vi "SPI.Get Address.vi"(10 "SPI.subSystem":T1=enum."DelayLine.MSB", 11 "ID":u8) -> (3 "Address":u16)   [LabVIEW 2018]
uses:
  SPI.SubSystem.ctl
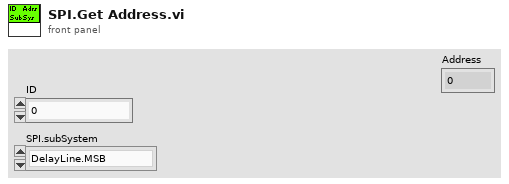
[diagram p1: front panel]
types:
  T1 = typedef "SPI.SubSystem.ctl" = enum8{"N/A", "DelayLine.MSB", "DelayLine.LSB", "Attenuation.dB", "Attenuation.DAC value", "SyncDetector.Offset", "SyncDetector.Comparator"}
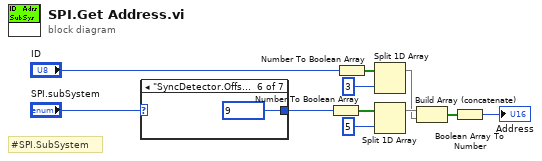
[diagram p0: block diagram]
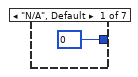
[diagram p2: hidden frame]
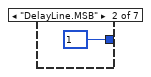
[diagram p3: hidden frame]
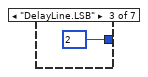
[diagram p4: hidden frame]
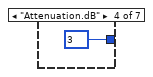
[diagram p5: hidden frame]
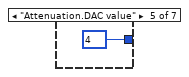
[diagram p6: hidden frame]
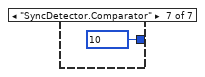
[diagram p7: hidden frame]
diagram:
  # "#SPI.SubSystem"
  n1 = case shown="\"SyncDetector.Offset\"" "SPI.subSystem" {
    tunnel: [0 1 2 3 4 9 10] -> w1
    frame "N/A", Default {
    }
    frame "DelayLine.MSB" {
    }
    frame "DelayLine.LSB" {
    }
    frame "Attenuation.dB" {
    }
    frame "Attenuation.DAC value" {
    }
    frame "SyncDetector.Offset" {
    }
    frame "SyncDetector.Comparator" {
    }
  }
  n2 = Number To Boolean Array(number=w1) -> (Boolean array=w9:bool[])
  n3 = Number To Boolean Array(number="ID") -> (Boolean array=w11:bool[])
  n4 = Split 1D Array(array=w11, index=3) -> (first subarray=w5:bool[])  [unwired: 1 out]
  n5 = Split 1D Array(array=w9, index=5) -> (first subarray=w7:bool[])  [unwired: 1 out]
  n6 = Build Array (concatenate)(w7, w5) -> (w6:bool[])
  n7 = Boolean Array To Number(Boolean array=w6) -> (number=→"Address":u16)
